vi "Motor wire organization.vi"(0 "Invert Motor 1 (Right Rear) (T)":bool=TRUE, 1 "Invert Motor 2 (Left Rear) (F)":bool, 3 "Invert Motor 3 (Right Front) (F)":bool, 4 "Invert Motor 4 (Left Front) (T)":bool=TRUE, 6 "Motor Speed 1 (Right Rear)":dbl(knob) scale=-1.0..1.0, 7 "Motor Speed 2 (Left Rear)":dbl(knob) scale=-1.0..1.0, 9 "Motor Speed 3 (Right Front)":dbl(knob) scale=-1.0..1.0, 10 "Motor Speed 4 (Left Front)":dbl(knob) scale=-1.0..1.0) -> (2 "Array of Motor Speeds":dbl[](array[numeric]))   [LabVIEW 2018]
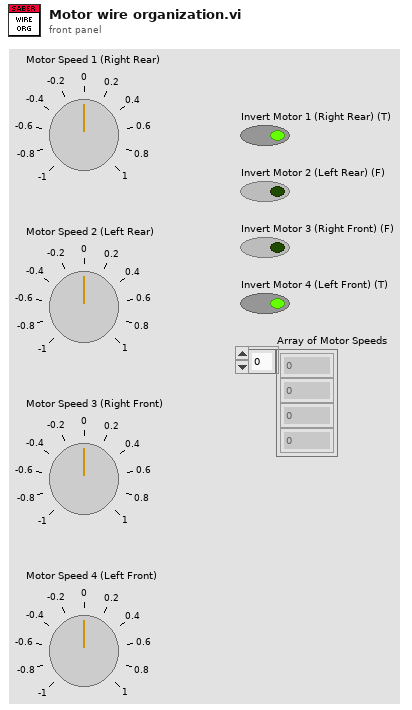
[diagram p1: front panel]
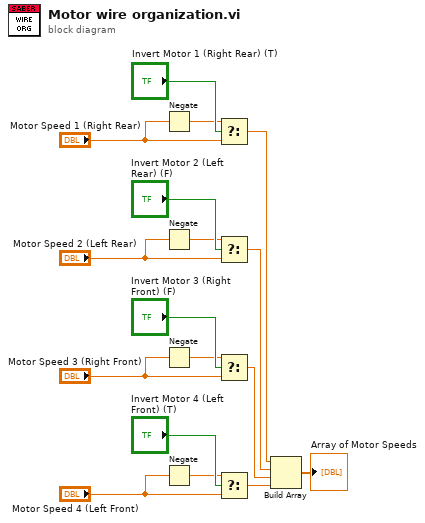
[diagram p0: block diagram]
diagram:
  n1 = Negate(x="Motor Speed 1 (Right Rear)") -> (-x=w12:dbl)
  n2 = Negate(x="Motor Speed 2 (Left Rear)") -> (-x=w11:dbl)
  n3 = Negate(x="Motor Speed 3 (Right Front)") -> (-x=w8:dbl)
  n4 = Negate(x="Motor Speed 4 (Left Front)") -> (-x=w6:dbl)
  n5 = Select(t=w12, s="Invert Motor 1 (Right Rear) (T)", f="Motor Speed 1 (Right Rear)") -> (s? t:f=w5:dbl)
  n6 = Select(t=w11, s="Invert Motor 2 (Left Rear) (F)", f="Motor Speed 2 (Left Rear)") -> (s? t:f=w4:dbl)
  n7 = Select(t=w8, s="Invert Motor 3 (Right Front) (F)", f="Motor Speed 3 (Right Front)") -> (s? t:f=w3:dbl)
  n8 = Select(t=w6, s="Invert Motor 4 (Left Front) (T)", f="Motor Speed 4 (Left Front)") -> (s? t:f=w2:dbl)
  n9 = Build Array(w5, w4, w3, w2) -> (→"Array of Motor Speeds":dbl[])
